vi "Process File Directory.vi"() -> (3 "Process File Directory":path)   [LabVIEW 2017]
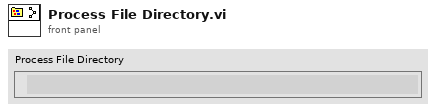
[diagram p1: front panel]
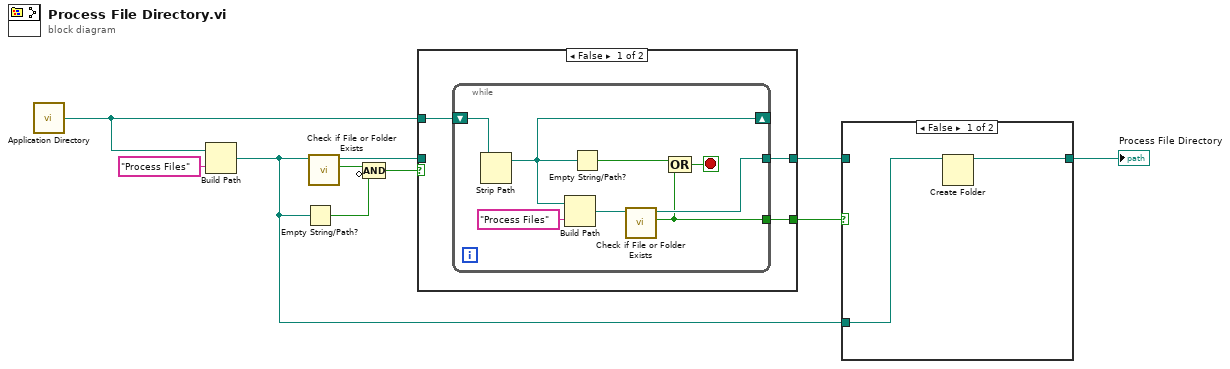
[diagram p0: block diagram]
diagram:
  n1 = call <vilib>:"Application Directory.vi"() -> ("Application Directory"=w5:path)
  n2 = Build Path(base path=w5, name or relative path="Process Files") -> (appended path=w2:path)
  n3 = Empty String/Path?(string/path=w2) -> (empty?=w8:bool)
  n4 = call <vilib>:"Check if File or Folder Exists.vi"("path"=w2) -> ("file or folder exists?"=w9:bool, "dup path"=w6:path)  [unwired: 8 in, 1 out]
  n5 = Compound Arithmetic op=AND(w9, invert w8) -> (w7:bool)
  n6 = case shown="False" w7 {
    selector: w7 -> [_ w22]
    tunnel: w6 -> [_ w23]
    tunnel: w5 -> [w13 _]
    tunnel: [w12 w23] -> w3
    tunnel: [w11 w22] -> w4
    frame False {
      n7 = while {
        shift-right: [w19] -> _
        shift-left: w13 -> [w21]
        tunnel: [w16] -> w12
        tunnel: [w14] -> w11
        stop <- w15 stop-if-true
        n8 = Strip Path(path=w21) -> (stripped path=w19:path)  [unwired: 1 out]
        n9 = Build Path(base path=w19, name or relative path="Process Files") -> (appended path=w18:path)
        n10 = Empty String/Path?(string/path=w19) -> (empty?=w17:bool)
        n11 = call <vilib>:"Check if File or Folder Exists.vi"("path"=w18) -> ("file or folder exists?"=w14:bool, "dup path"=w16:path)  [unwired: 8 in, 1 out]
        n12 = Compound Arithmetic op=OR(w17, w14) -> (w15:bool)
      }
    }
    frame True {
    }
  }
  n13 = case shown="False" w4 {
    tunnel: w3 -> [_ w26]
    tunnel: w2 -> [w25 _]
    tunnel: [w24 w26] -> w1
    frame False {
      n14 = Create Folder(path (use dialog)=w25) -> (created path=w24:path)  [unwired: 2 in, 2 out]
    }
    frame True {
    }
  }
  "Process File Directory" <- w1
